vi "File Tracker.vi"(5 "Gas":string="#GasID=", 7 "Command":string, 8 "error in (no error)":errorcluster, 9 "Blob":u8[](array[numeric]), 10 "Result":T1={"Gas Counter"=0, "Filter Counter"=0, "ADC Samples"=[], "Gas Timeout"=0, "Notes"="Success", "Moisture"=0.1625, "PPM"=1.0, "Mean"=197500.0, "STD"=1200.0, "Gas"="N", "Pressure"=12.0, "Temp"=35.0, "Samples"=20, "Filter"=1, "Phase"=60.0}, 11 "Readings":cluster{"mean":dbl, "standard deviation":dbl}[](array[cluster])=[{"mean"=3352.9600000000005, "standard deviation"=988.6516974029721}, {"mean"=3138.5999999999995, "standard deviation"=1141.3182378285208}, {"mean"=2395.825, "standard deviation"=935.6369388015845}, {"mean"=2679.8450000000003, "standard deviation"=848.7435378415424}, {"mean"=2575.6899999999996, "standard deviation"=704.8861337517965}, {"mean"=3508.55, "standard deviation"=1511.7860039260408}, {"mean"=3222.18, "standard deviation"=1340.8528080624246}, {"mean"=3221.015, "standard deviation"=2308.8843542150157}, {"mean"=2810.255, "standard deviation"=867.7062615661541}]) -> (0 "error out":errorcluster, 3 "File Contents":string)   [LabVIEW 2015]
uses:
  Controls/Test Info.ctl
panel:
  out "appended path":path
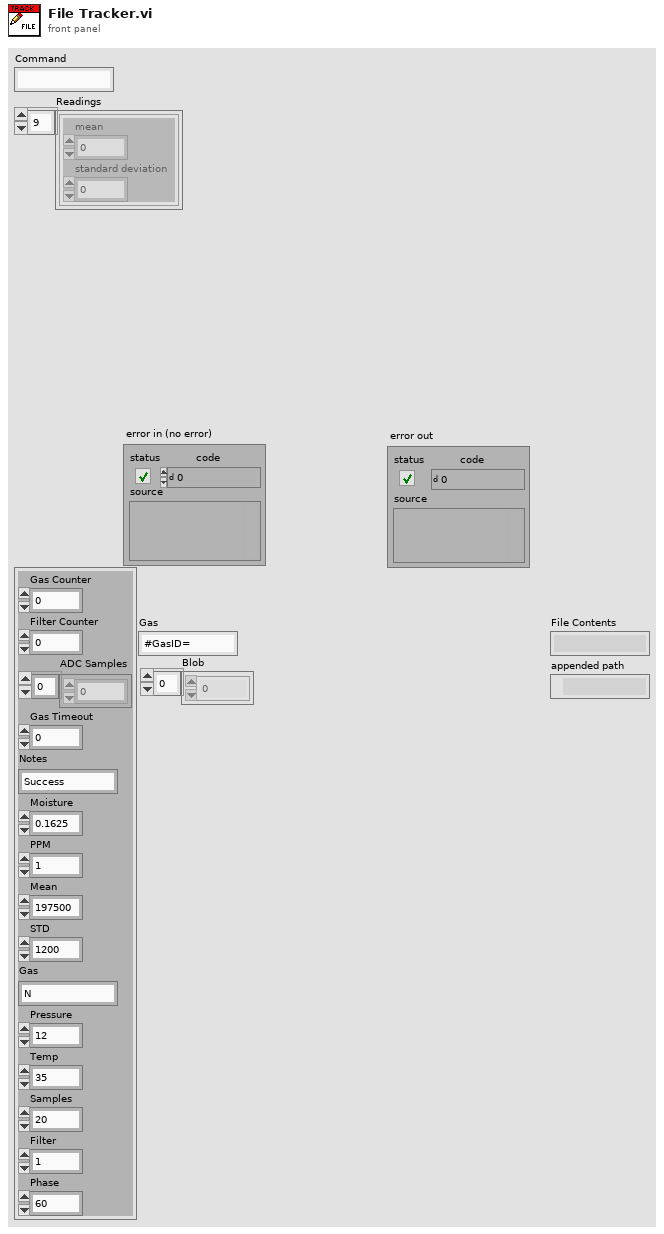
[diagram p1: front panel]
types:
  T1 = typedef "Test Info.ctl" = cluster{"Gas Counter":u16, "Filter Counter":u16, "ADC Samples":dbl[], "Gas Timeout":u16, "Notes":string, "Moisture":dbl, "PPM":dbl, "Mean":dbl, "STD":dbl, "Gas":string, "Pressure":dbl, "Temp":dbl, "Samples":u16, "Filter":u8, "Phase":dbl}
  T2 = enum16{"open", "replace", "create", "open or create", "replace or create", "replace or create with confirmation"}
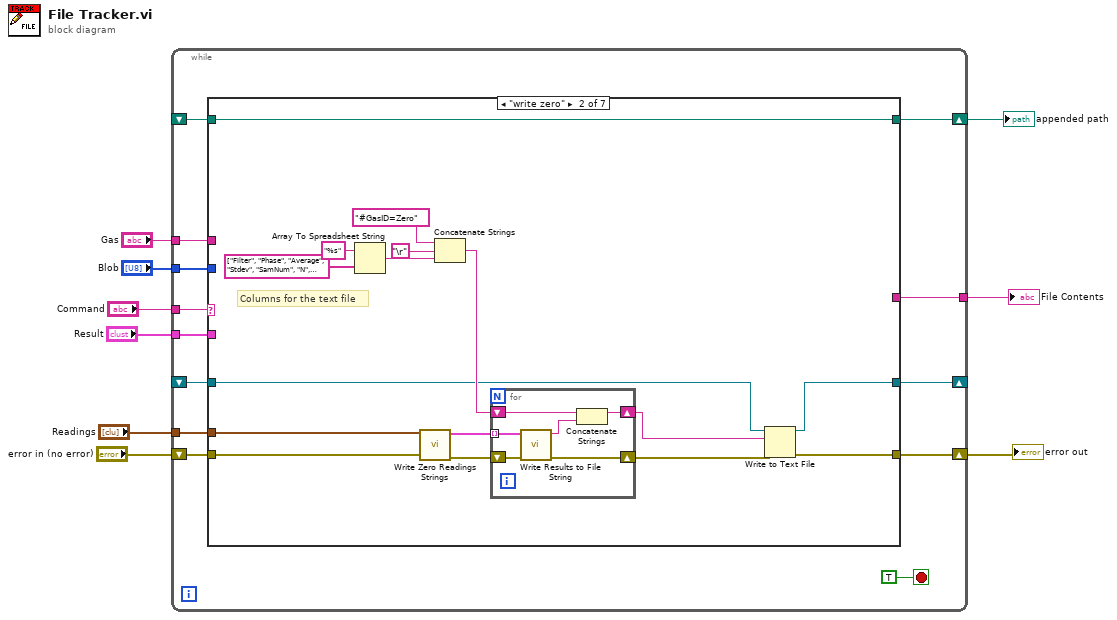
[diagram p0: block diagram]
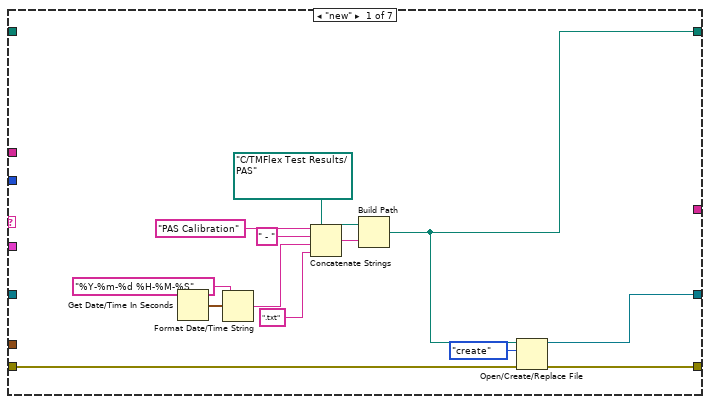
[diagram p2: hidden frame]
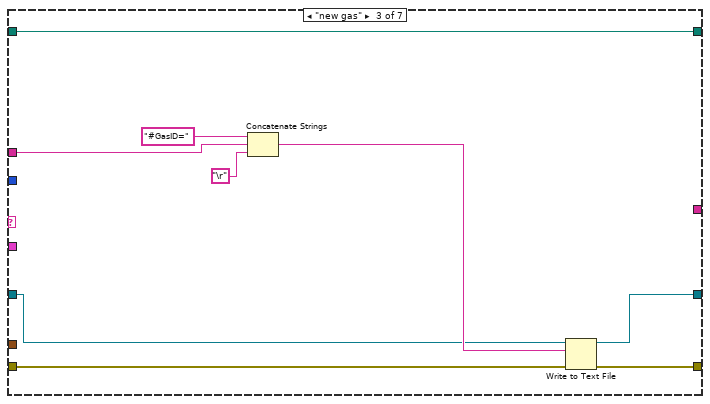
[diagram p3: hidden frame]
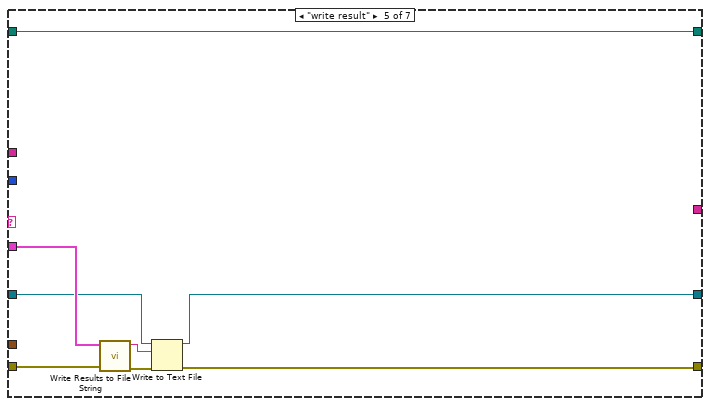
[diagram p5: hidden frame]
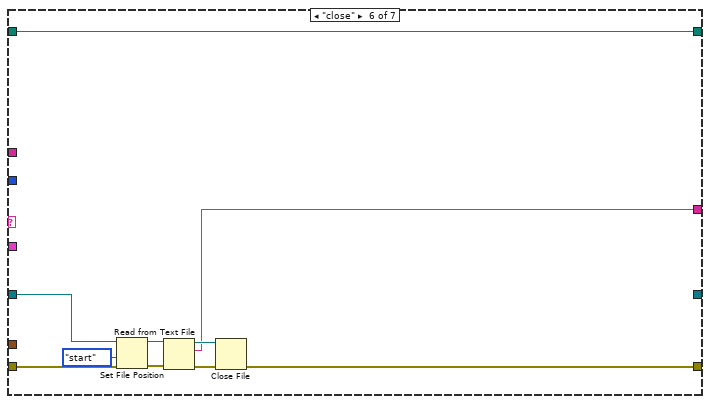
[diagram p6: hidden frame]
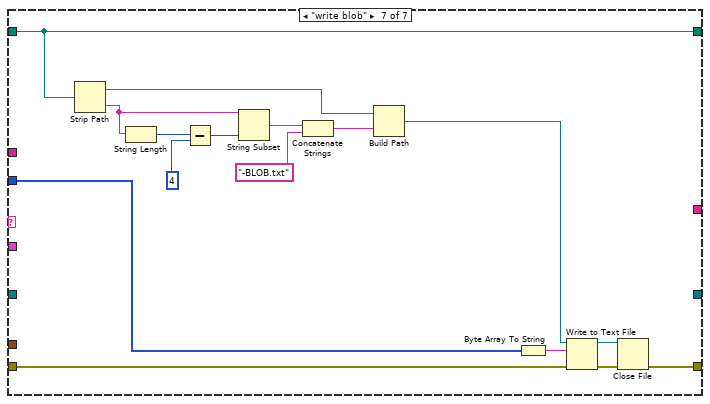
[diagram p7: hidden frame]
diagram:
  n1 = while {
    tunnel: "Command" -> [w21]
    shift-right: [w19] -> w7
    shift-left: "error in (no error)" -> [w20]
    tunnel: "Readings" -> [w18]
    shift-right: [w17] -> _
    shift-left: _ -> [w16]
    tunnel: "Result" -> [w15]
    tunnel: [w14] -> w4
    tunnel: "Gas" -> [w13]
    shift-right: [w12] -> w2
    shift-left: _ -> [w11]
    tunnel: "Blob" -> [w10]
    stop <- TRUE stop-if-true
    n2 = case shown="\"write zero\"" w21 {
      tunnel: w20 -> [w27 w50 w64 w69 w77 w82 w103]
      tunnel: [w26 w51 w66 w69 w71 w87 w90] -> w19
      tunnel: w18 -> [_ w49 _ _ _ _ _]
      tunnel: [w23 w38 w65 w68 w72 _ _] -> w17
      tunnel: w16 -> [_ w36 w59 w68 w73 w83 _]
      tunnel: w15 -> [_ _ _ _ w76 _ _]
      tunnel: [_ _ _ _ _ w84 _] -> w14
      tunnel: w13 -> [_ _ w62 _ _ _ _]
      tunnel: [w24 w37 w58 w67 w70 w78 w94] -> w12
      tunnel: w11 -> [_ w37 w58 w67 w70 w78 w94]
      tunnel: w10 -> [_ _ _ _ _ _ w88]
      frame "new" {
        n3 = Get Date/Time In Seconds() -> (seconds since 1Jan1904=w35:timestamp)
        n4 = Format Date/Time String(time format string (%c)="%Y-%m-%d %H-%M-%S", seconds (now)=w35) -> (date/time string=w33:string)  [unwired: 1 in]
        n5 = Concatenate Strings("PAS Calibration" ("string"), " - " ("string"), w33, ".txt" ("string")) -> (w29:string)
        n6 = Build Path(base path=path "C:/TMFlex Test Results/PAS" ("path"), name or relative path=w29) -> (appended path=w24:path)
        n7 = Open/Create/Replace File(file path (use dialog)=w24, error in=w27, operation (0:open)=T2."create") -> (refnum out=w23:refnum<file>, error out=w26:errorcluster)  [unwired: 3 in, 1 out]
      }
      frame "write zero" {
        # "Columns for the text file"
        n8 = Array To Spreadsheet String(array=string[] ["Filter", "Phase", "Average", "Stdev", "SamNum", "N", "CH4", "C2H6", "C2H4", "C2H2", "CO", "CO2", "H2O", "O2", "H2", "C3H8", "C3H6", "PASTemp", "PASPressure", "Notes"], 3:"%s" ("format string")) -> (spreadsheet string=w40:string)  [unwired: 1 in]
        n9 = call "Write Zero Readings Strings.vi"("error in (no error)"=w50, "Zero Readings"=w49) -> ("error out"=w48:errorcluster, "Results"=w47:T1[])  [unwired: 8 in]
        n10 = Concatenate Strings("#GasID=Zero", "\r", w40) -> (w39:string)
        n11 = for {
          tunnel: w47 -> [w56] mode=indexing
          shift-right: [w55] -> w46
          shift-left: w48 -> [w57]
          shift-right: [w52] -> w45
          shift-left: w39 -> [w54]
          n12 = call "Write Results to File String.vi"("error in (no error)"=w57, "Result"=w56) -> ("error out"=w55:errorcluster, "spreadsheet string"=w53:string)  [unwired: 8 in]
          n13 = Concatenate Strings(w54, w53) -> (w52:string)
        }
        n14 = Write to Text File(file (use dialog)=w36, text=w45, error in=w46) -> (refnum out=w38:refnum<file>, error out=w51:errorcluster)  [unwired: 1 in, 1 out]
      }
      frame "new gas" {
        n15 = Concatenate Strings("#GasID=", w62, "\r") -> (w60:string)
        n16 = Write to Text File(file (use dialog)=w59, text=w60, error in=w64) -> (refnum out=w65:refnum<file>, error out=w66:errorcluster)  [unwired: 1 in, 1 out]
      }
      frame Default {
      }
      frame "write result" {
        n17 = call "Write Results to File String.vi"("error in (no error)"=w77, "Result"=w76) -> ("error out"=w75:errorcluster, "spreadsheet string"=w74:string)  [unwired: 8 in]
        n18 = Write to Text File(file (use dialog)=w73, text=w74, error in=w75) -> (refnum out=w72:refnum<file>, error out=w71:errorcluster)  [unwired: 1 in, 1 out]
      }
      frame "close" {
        n19 = Set File Position(refnum=w83, from (0:start)=enum16{"start", "end", "current"}."start", error in=w82) -> (refnum out=w80:refnum<file>, error out=w81:errorcluster)  [unwired: 1 in]
        n20 = Read from Text File(file (use dialog)=w80, error in=w81) -> (refnum out=w85:refnum<file>, text=w84:string, error out=w86:errorcluster)  [unwired: 2 in, 1 out]
        n21 = Close File(refnum=w85, error in=w86) -> (error out=w87:errorcluster)  [unwired: 1 out]
      }
      frame "write blob" {
        n22 = Strip Path(path=w94) -> (stripped path=w96:path, name=w102:string)
        n23 = String Length(string=w102) -> (length=w101:i32)
        n24 = Subtract(x=w101, y=4) -> (x-y=w99:i32)
        n25 = String Subset(string=w102, length (rest)=w99) -> (substring=w98:string)  [unwired: 1 in]
        n26 = Concatenate Strings(w98, "-BLOB.txt" ("string")) -> (w95:string)
        n27 = Build Path(base path=w96, name or relative path=w95) -> (appended path=w93:path)
        n28 = Byte Array To String(unsigned byte array=w88) -> (string=w89:string)
        n29 = Write to Text File(file (use dialog)=w93, text=w89, error in=w103) -> (refnum out=w91:refnum<file>, error out=w92:errorcluster)  [unwired: 1 in, 1 out]
        n30 = Close File(refnum=w91, error in=w92) -> (error out=w90:errorcluster)  [unwired: 1 out]
      }
    }
  }
  "error out" <- w7
  "File Contents" <- w4
  "appended path" <- w2
